vi "GetEnumValue.vi"(2 "error in (no error)":errorcluster, 3 "Feature Name":string, 4 "IGxDevice":refnum<k24>) -> (0 "error out":errorcluster, 1 "Enum Value":string)   [LabVIEW 2013, in "GxLVlib.lvlib"]
uses:
  GxLVlib.lvlib
  F:/GxILibrary/Labview/trunk/private/dev/src/C#/x86/GxLVLib/dll/GxIAPINET.dll
  private/dev/src/C#/x86/GxLVLib/dll/GxIAPINET.dll
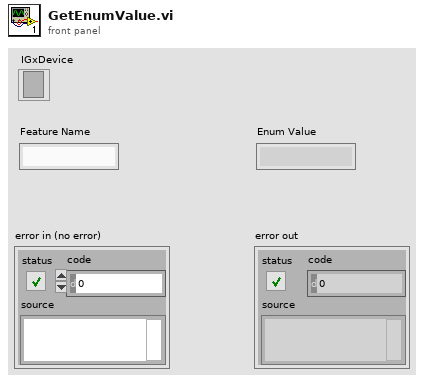
[diagram p1: front panel]
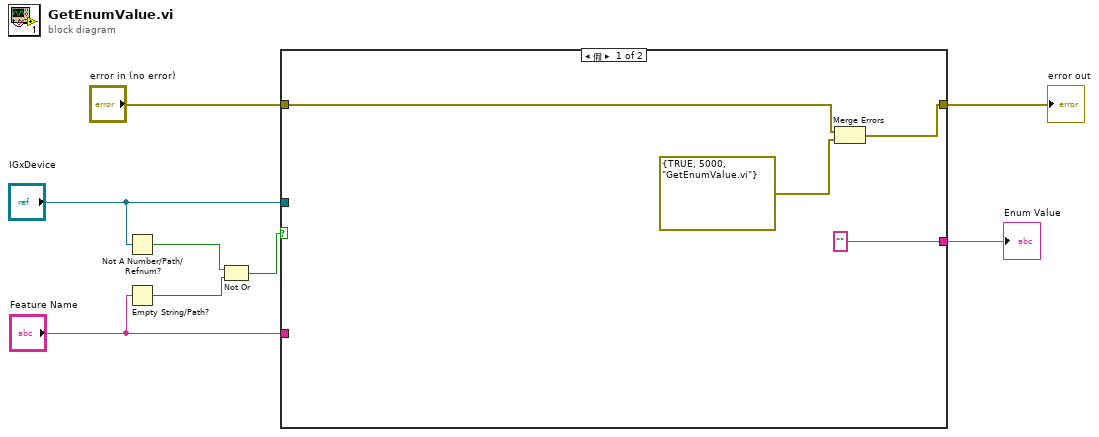
[diagram p0: block diagram]
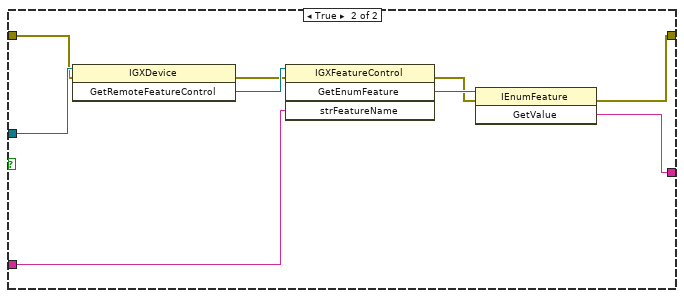
[diagram p2: hidden frame]
diagram:
  n1 = Not A Number/Path/Refnum?(number/path/refnum="IGxDevice") -> (NaN/Path/Refnum?=w8:bool)
  n2 = Empty String/Path?(string/path="Feature Name") -> (empty?=w7:bool)
  n3 = Not Or(1:w7, 2:w8) -> (0:w6:bool)
  n4 = case shown="假" w6 {
    tunnel: "error in (no error)" -> [w10 w20]
    tunnel: [w9 w13] -> w4
    tunnel: "IGxDevice" -> [_ w21]
    tunnel: "Feature Name" -> [_ w17]
    tunnel: ["" w14] -> w1
    frame False {
      n5 = Merge Errors(w10, errorcluster {TRUE, 5000, "GetEnumValue.vi"}) -> (w9:errorcluster)
    }
    frame True {
      n6 = invoke class="IGXDevice" method="GetRemoteFeatureControl"(reference=w21, error in=w20) -> (error out=w18:errorcluster, "GetRemoteFeatureControl"=w19:refnum<k24>)  [unwired: 1 in, 1 out]
      n7 = invoke class="IGXFeatureControl" method="GetEnumFeature"(reference=w19, error in=w18, "strFeatureName"=w17) -> (error out=w15:errorcluster, "GetEnumFeature"=w16:refnum<k24>)  [unwired: 1 in, 2 out]
      n8 = invoke class="IEnumFeature" method="GetValue"(reference=w16, error in=w15) -> (error out=w13:errorcluster, "GetValue"=w14:string)  [unwired: 1 in, 1 out]
    }
  }
  "error out" <- w4
  "Enum Value" <- w1
